vi "BRig_generic_pathCreate_pathInput.vi"(8 "input_error":errorcluster, 11 "input_filePath":path) -> (0 "output_error":errorcluster, 3 "output_filePath":path)   [LabVIEW 2014]
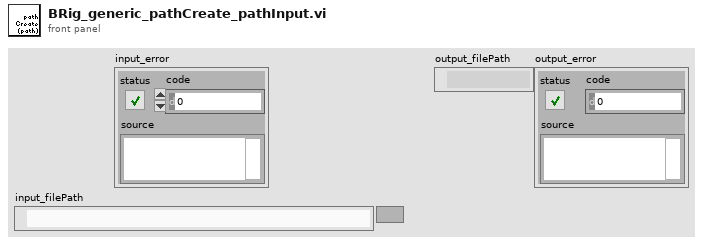
[diagram p1: front panel]
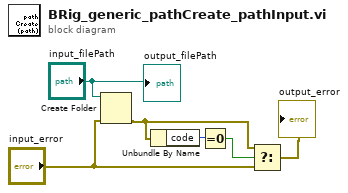
[diagram p0: block diagram]
diagram:
  n1 = Create Folder(path (use dialog)="input_filePath", error in="input_error") -> (error out=w2:errorcluster)  [unwired: 1 in, 2 out]
  n2 = Unbundle By Name(w2) -> ("code"=w6:i32)
  n3 = Equal To 0?(x=w6) -> (x = 0?=w5:bool)
  n4 = Select(t=w2, s=w5, f="input_error") -> (s? t:f=→"output_error":errorcluster)
  "output_filePath" <- "input_filePath"
